vi "_TreeItem.Property.Get.Dictionary.Read.vi"(8 "error in (no error)":errorcluster, 9 "Keys":string[](array[string]), 10 "Type":string, 11 "DictionaryProperty":refnum<k24>) -> (0 "error out":errorcluster, 2 "Dictionary Variant":variant, 3 "DictionaryProperty out":refnum<k24>)   [LabVIEW 2016, in "Advanced System Definition.lvlib"]
uses:
  SysDef API/Advanced System Definition.lvlib
  NationalInstruments.VeriStand.SystemStorage
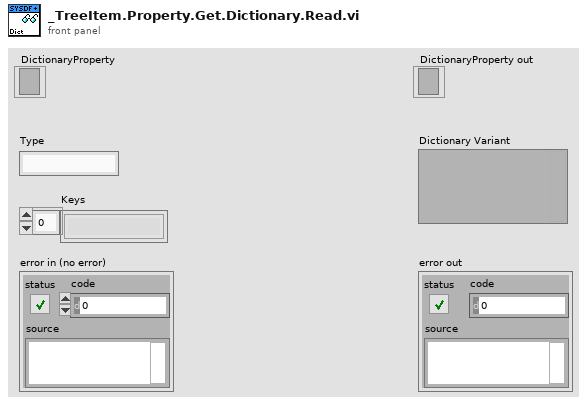
[diagram p1: front panel]
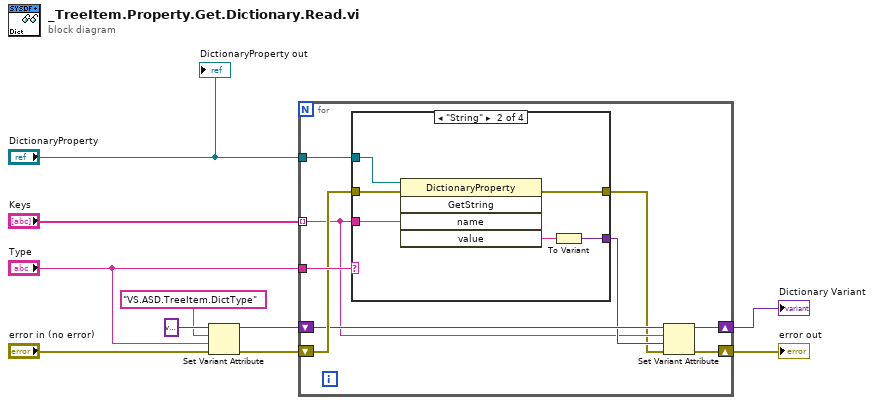
[diagram p0: block diagram]
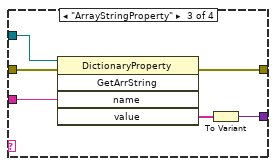
[diagram p3: hidden frame]
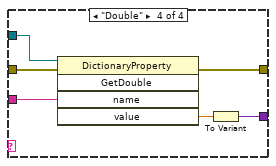
[diagram p4: hidden frame]
diagram:
  n1 = Set Variant Attribute(Variant=variant, name="VS.ASD.TreeItem.DictType", value="Type", error in="error in (no error)") -> (Variant out=w1:variant, error out=w2:errorcluster)  [unwired: 1 out]
  n2 = for {
    tunnel: "Type" -> [w19]
    tunnel: "DictionaryProperty" -> [w18]
    tunnel: "Keys" -> [w14] mode=indexing
    shift-right: [w11] -> w9
    shift-left: w2 -> [w17]
    shift-right: [w13] -> w7
    shift-left: w1 -> [w16]
    n3 = case shown="\"String\"" w19 {
      tunnel: w18 -> [_ w26 w32 w38]
      tunnel: w17 -> [w20 w25 w31 w37]
      tunnel: [w20 w24 w30 w36] -> w12
      tunnel: w14 -> [_ w23 w29 w35]
      tunnel: [_ w21 w27 w33] -> w15
      frame Default {
      }
      frame "String" {
        n4 = invoke class="DictionaryProperty" method="GetString"(reference=w26, error in=w25, "name"=w23) -> (error out=w24:errorcluster, "value"=w22:string)  [unwired: 2 in, 3 out]
        n5 = To Variant(anything=w22) -> (Variant=w21:variant)
      }
      frame "ArrayStringProperty" {
        n6 = invoke class="DictionaryProperty" method="GetArrString"(reference=w32, error in=w31, "name"=w29) -> (error out=w30:errorcluster, "value"=w28:string[])  [unwired: 2 in, 3 out]
        n7 = To Variant(anything=w28) -> (Variant=w27:variant)
      }
      frame "Double" {
        n8 = invoke class="DictionaryProperty" method="GetDouble"(reference=w38, error in=w37, "name"=w35) -> (error out=w36:errorcluster, "value"=w34:dbl)  [unwired: 2 in, 3 out]
        n9 = To Variant(anything=w34) -> (Variant=w33:variant)
      }
    }
    n10 = Set Variant Attribute(Variant=w16, name=w14, value=w15, error in=w12) -> (Variant out=w13:variant, error out=w11:errorcluster)  [unwired: 1 out]
  }
  "Dictionary Variant" <- w7
  "error out" <- w9
  "DictionaryProperty out" <- "DictionaryProperty"
